vi "Execute CleanUp Step.vi"(8 "error in (no error)":errorcluster, 9 "result allocation in":T1, 10 "parameters":T1, 11 "Sequencer Module runtime in":refnum<class "Sequencer Module runtime.lvclass">) -> (0 "error out":errorcluster, 1 "results":T1, 2 "parameter allocation":T1, 3 "Sequencer Module runtime out":refnum<class "Sequencer Module runtime.lvclass">)   [LabVIEW 2015, in "Sequencer Module runtime.lvclass"]
uses:
  Sequencer Module runtime.lvclass
  <vilib>/NI/Tag Bus/table/data table.ctl
  Sequencer Module runtime.lvclass/Sequencer Module runtime.ctl
  classes/Sequence/Execution/Sequence.lvclass
  classes/Step/Execution/Step.lvclass
  <vilib>/NI/Tag Bus/table/data table.lvlib
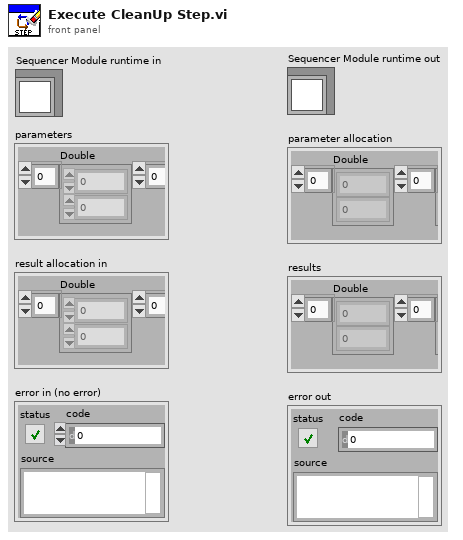
[diagram p1: front panel]
types:
  T1 = typedef "tag bus.lvlib/data table.lvlib/data table.ctl" = cluster{"Double":dbl[], "Single":sgl[], "I64":i64[], "I32":i32[], "I16":i16[], "I8":i8[], "U64":u64[], "U32":u32[], "U16":u16[], "U8":u8[], "Boolean":bool[], "String":string[], "Array of Double":cluster{"DBL Array":dbl[]}[], "Array of Single":cluster{"SGL Array":sgl[]}[], "Array of I64":cluster{"I64 Array":i64[]}[], "Array of I32":cluster{"I32 Array":i32[]}[], "Array of I16":cluster{"I16 Array":i16[]}[], "Array of I8":cluster{"I8 Array":i8[]}[], "Array of U64":cluster{"U64 Array":u64[]}[], "Array of U32":cluster{"U32 Array":u32[]}[], "Array of U16":cluster{"U16 Array":u16[]}[], "Array of U8":cluster{"U8 Array":u8[]}[], "Array of Boolean":cluster{"Boolean Array":bool[]}[], "Array of String":cluster{"String Array":string[]}[]}
  T2 = typedef "Step.lvclass/StepState.ctl" = cluster{"Step State":T3, "Flow Control":T4, "Jump Index":i32, "Done":bool}
  T3 = typedef "Step.lvclass/Step Status.ctl" = enum16{"Start", "Passed", "Failed", "Error", "Done", "Terminated", "Skipped", "Running"}
  T4 = typedef "Step.lvclass/Step Flow Control.ctl" = enum16{"Next Step", "Jump"}
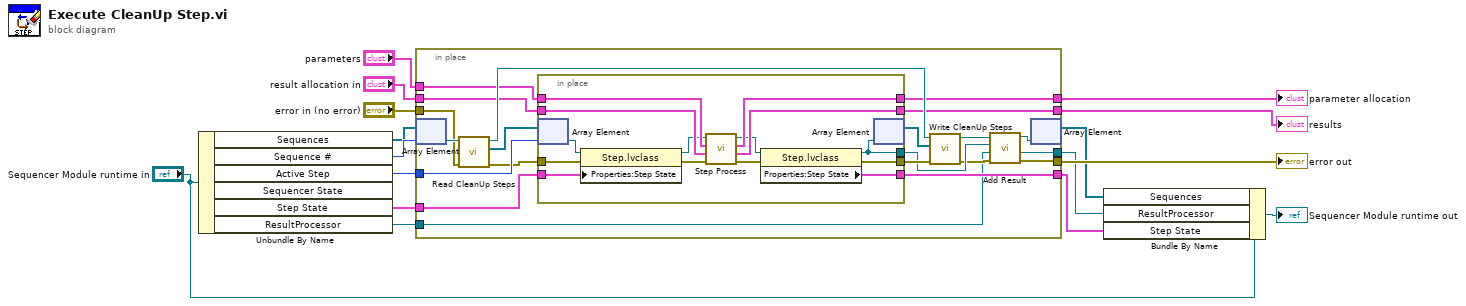
[diagram p0: block diagram]
diagram:
  n1 = Unbundle By Name("Sequencer Module runtime in") -> ("Sequences"=w11:refnum<class "Sequence.lvclass">[], "Sequence #"=w12:i32, "Active Step"=w13:i32, "Step State"=w14:T2, "ResultProcessor"=w3:refnum<class "ResultProcessor.lvclass">)  [unwired: 1 out]
  n2 = in-place {
    in-place-border: w13 -> [w37]
    in-place-border: "error in (no error)" -> [w32]
    in-place-border: [w21] -> w16
    in-place-border: [w29] -> w2
    in-place-border: w14 -> [w28]
    in-place-border: "parameters" -> [w27]
    in-place-border: [w26] -> w7
    in-place-border: "result allocation in" -> [w25]
    in-place-border: [w24] -> w9
    in-place-border: w3 -> [w18]
    in-place-border: [w17] -> w1
    n3 = in-place-array #1(w11, w12) -> (w36:refnum<class "Sequence.lvclass">)
    n4 = call-dynamic "Read CleanUp Steps.vi"("error in (no error)"=w32, "Sequence in"=w36) -> ("error out"=w31:errorcluster, "CleanUp Steps"=w35:refnum<class "Step.lvclass">[], "Sequence out"=w33:refnum<class "Sequence.lvclass">)  [unwired: 7 in]
    n5 = in-place {
      in-place-border: w31 -> [w44]
      in-place-border: [w39] -> w30
      in-place-border: [w41] -> w29
      in-place-border: w28 -> [w47]
      in-place-border: w27 -> [w51]
      in-place-border: [w50] -> w26
      in-place-border: w25 -> [w49]
      in-place-border: [w48] -> w24
      in-place-border: [w38] -> w20
      n6 = in-place-array #2(w35, w37) -> (w46:refnum<class "Step.lvclass">)
      n7 = property class="Step.lvclass"(reference=w46, error in=w44, "Properties:Step State"=w47) -> (reference out=w45:refnum<class "Step.lvclass">, error out=w43:errorcluster)
      n8 = call-dynamic "Step Process.vi"("error in (no error)"=w43, "result allocation"=w49, "parameters"=w51, "Step in"=w45) -> ("error out"=w40:errorcluster, "results"=w48:T1, "parameter allocation"=w50:T1, "Step out"=w42:refnum<class "Step.lvclass">)  [unwired: 4 in]
      n9 = property class="Step.lvclass"(reference=w42, error in=w40) -> (reference out=w38:refnum<class "Step.lvclass">, error out=w39:errorcluster, "Properties:Step State"=w41:T2)
      n10 = in-place-array #2(w38) -> (w34:refnum<class "Step.lvclass">[])  [unwired: 1 out]
    }
    n11 = call-dynamic "Write CleanUp Steps.vi"("error in (no error)"=w30, "CleanUp Steps"=w34, "Sequence in"=w33) -> ("error out"=w19:errorcluster, "Sequence out"=w23:refnum<class "Sequence.lvclass">)  [unwired: 7 in]
    n12 = call-dynamic "Add Result.vi"("error in (no error)"=w19, "ResultProcessor in"=w18, "Step"=w20, "Sequence in"=w23) -> ("error out"=w21:errorcluster, "ResultProcessor out"=w17:refnum<class "ResultProcessor.lvclass">, "Sequence out"=w22:refnum<class "Sequence.lvclass">)  [unwired: 5 in]
    n13 = in-place-array #1(w22) -> (w5:refnum<class "Sequence.lvclass">[])  [unwired: 1 out]
  }
  "error out" <- w16
  "results" <- w9
  "parameter allocation" <- w7
  n14 = Bundle By Name(cluster="Sequencer Module runtime in", "Sequences"=w5, "ResultProcessor"=w1, "Step State"=w2) -> (→"Sequencer Module runtime out":refnum<class "Sequencer Module runtime.lvclass">)
